vi "SwerveDriveRotate.vi"(7 "Trigger Axes":cluster{"Left":dbl, "Right":dbl}, 8 "error in (no error)":errorcluster, 9 "Center of Rotation Joystick Axes":cluster{"X":dbl, "Y":dbl}, 10 "Strafe Joystick Axes":cluster{"X":dbl, "Y":dbl}, 11 "Angle (degrees; 0 = right)":dbl) -> (0 "error out":errorcluster)   [LabVIEW 2014]
uses:
  Robot Global Data.vi
panel:
  out "FL":dbl(slide) scale=-1.0..1.0
  out "FR":dbl(slide) scale=-1.0..1.0
  out "RL":dbl(slide) scale=-1.0..1.0
  out "RR":dbl(slide) scale=-1.0..1.0
  out "RL":dbl(knob) scale=3.1416..-3.1416
  out "RR":dbl(knob) scale=3.1416..-3.1416
  out "FR":dbl(knob) scale=3.1416..-3.1416
  out "FL":dbl(knob) scale=3.1416..-3.1416
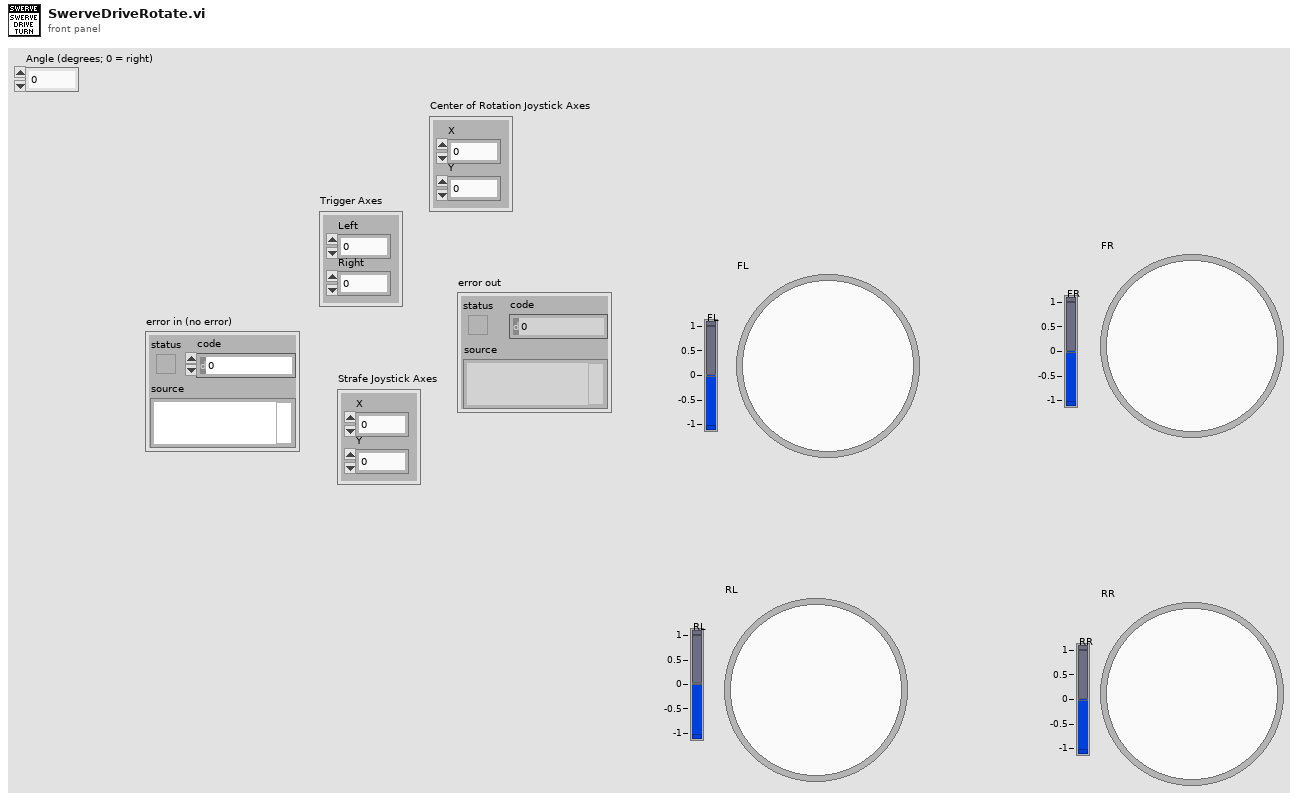
[diagram p1: front panel]
types:
  T1 = typedef "WPI_MotorControlDeviceRef.ctl" = cluster{"DeviceStatus":errorcluster, "Type":T2, "PWM":cluster{"Controller":T3, "PWM Channel":T4, "DeadBand":T5}, "CAN":cluster{"Device Number":u8, "Control Mode":T6, "Semaphore":T7, "Max Vout":dbl, "TalonSRX Control Mode":T8}, "Invert":bool, "TransformRef":T9, "InvTransformRef":T9}
  T2 = typedef "WPI_MotorControlType.ctl" = enum16{"PWM", "CAN", "CANTalonSRX"}
  T3 = typedef "FPGA_TypedefDigitalModule.ctl" = enum16{"Controller 1"}
  T4 = typedef "FPGA_DIOPWMChannel.ctl" = enum8{"PWM 0", "PWM 1", "PWM 2", "PWM 3", "PWM 4", "PWM 5", "PWM 6", "PWM 7", "PWM 8", "PWM 9", "PWM MXP 0", "PWM MXP 1", "PWM MXP 2", "PWM MXP 3", "PWM MXP 4", "PWM MXP 5", "PWM MXP 6", "PWM MXP 7", "PWM MXP 8", "PWM MXP 9", "Invalid"}
  T5 = typedef "WPI_PWMDeadband.ctl" = cluster{"Name":string, "maxPositivePwm":i32, "minPositivePwm":i32, "centerPwm":i32, "maxNegativePwm":i32, "minNegativePwm":i32, "angularRange":u16}
  T6 = typedef "WPI_CANJaguar_ControlMode.ctl" = enum8{"Percent VBus", "Current", "Speed", "Position", "Voltage"}
  T7 = typedef "Semaphore RefNum" = refnum<k1>
  T8 = typedef "WPI_CANTalonSRX_APIControlMode.ctl" = enum8{"Percent VBus", "Speed", "Position", "Slave", "Unchanged / Invalid"}
  T9 = typedef "WPI_PWMTransform_ConPane.ctl" = refnum<vi>
  T10 = typedef "WPI_CANTalonSRX_GlobalStatus.ctl" = cluster{"Applied Throttle":dbl, "Module Enabled":bool, "CAN Error":errorcluster, "Closed Loop Error":dbl, "Forward Limit Switch Closed":bool, "Reverse Limit Switch Closed":bool, "Sensor Position":dbl, "Sensor Velocity":dbl, "Current":dbl, "Sticky Fault - Over Temp":bool, "Sticky Fault - Under Voltage":bool, "Sticky Fault - Forward Limit":bool, "Sticky Fault - Reverse Limit":bool, "Sticky Fault - Forward Soft Limit":bool, "Sticky Fault - Reverse Soft Limit":bool, "Brake is Enabled":bool, "Encoder Position":dbl, "Encoder Velocity":dbl, "Encoder Index Count":dbl, "Encoder A Pin State":bool, "Encoder B Pin State":bool, "Encoder Index Pin State":bool, "Analog In":dbl, "Analog In Velocity":dbl, "Temperature (C)":dbl, "Battery Voltage":dbl}
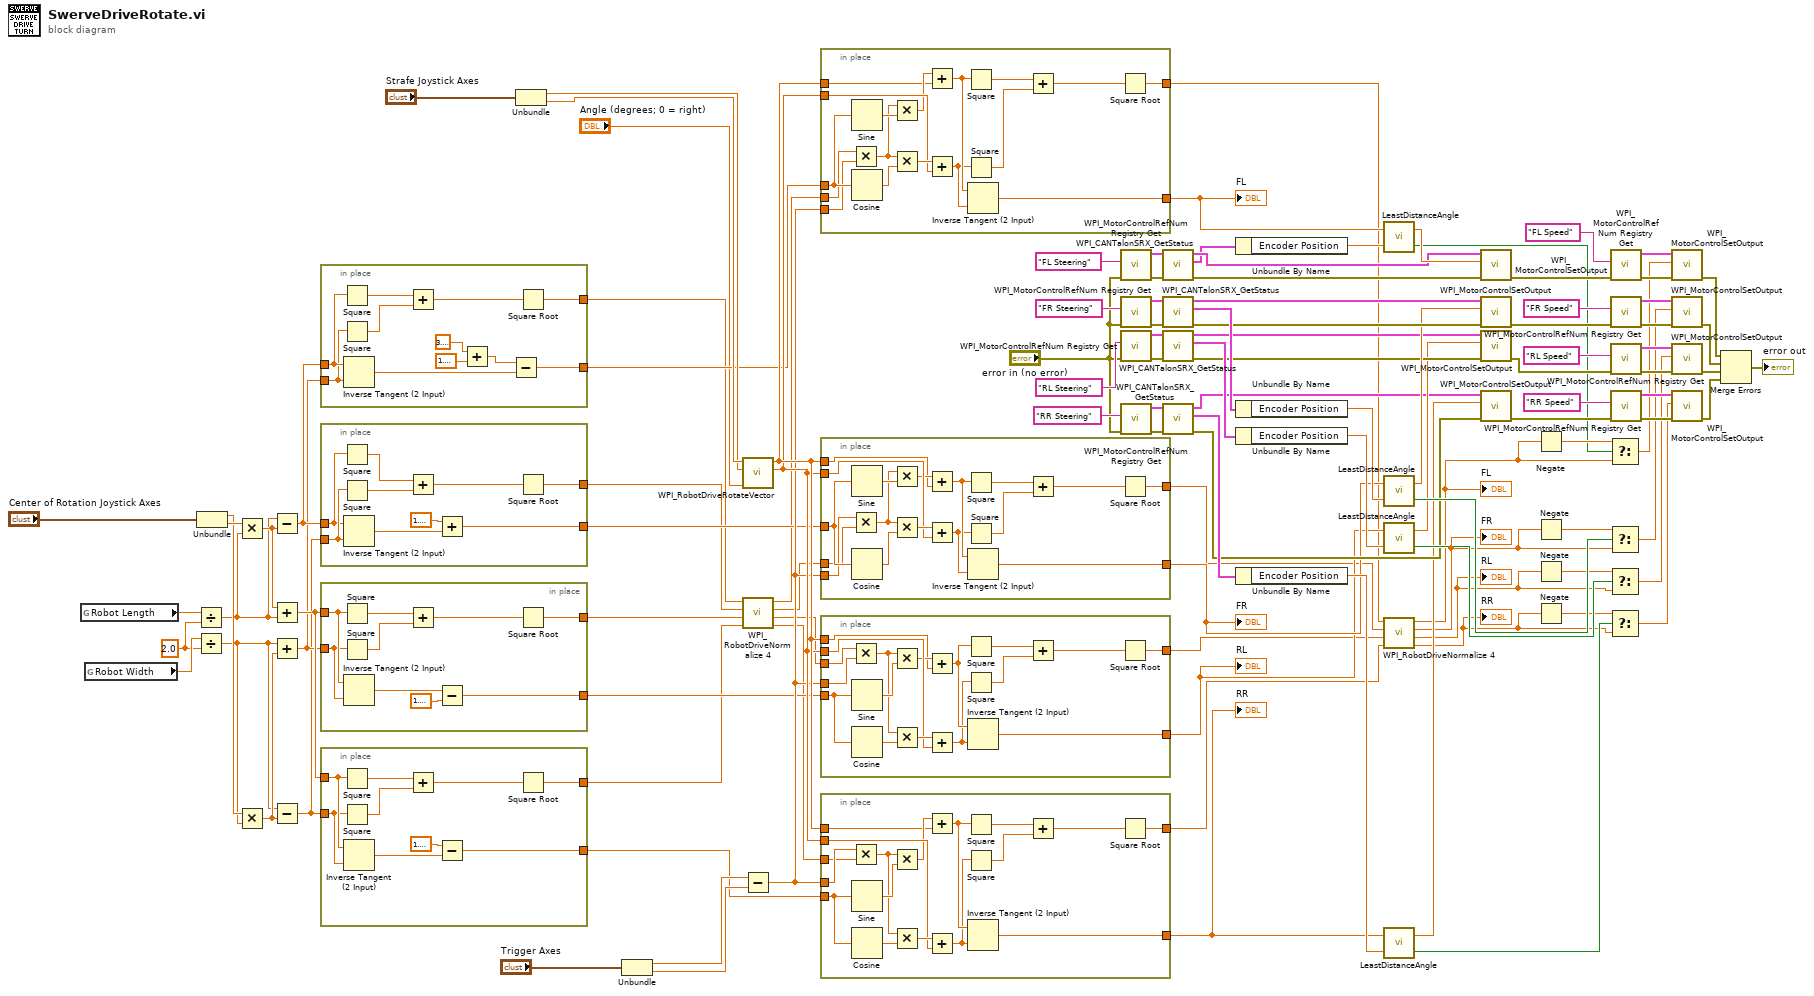
[diagram p0: block diagram]
diagram:
  w34 = 2.0 ("y")
  n1 = global read "Robot Global Data.vi" "Robot Length"() -> (w36:dbl)
  n2 = global read "Robot Global Data.vi" "Robot Width"() -> (w35:dbl)
  n3 = Divide(x=w36, y=w34) -> (x/y=w29:dbl)
  n4 = Divide(x=w35, y=w34) -> (x/y=w28:dbl)
  n5 = Unbundle("Center of Rotation Joystick Axes") -> ("X"=w32:dbl, "Y"=w33:dbl)
  n6 = Multiply(x=w33, y=w29) -> (x*y=w30:dbl)
  n7 = Multiply(x=w32, y=w28) -> (x*y=w31:dbl)
  n8 = Subtract(x=w29, y=w30) -> (x-y=w23:dbl)
  n9 = Add(x=w30, y=w29) -> (x+y=w22:dbl)
  n10 = Add(x=w28, y=w31) -> (x+y=w21:dbl)
  n11 = Subtract(x=w28, y=w31) -> (x-y=w19:dbl)
  n12 = in-place {
    in-place-border: [w125] -> w14
    in-place-border: w23 -> [w117]
    in-place-border: w21 -> [w116]
    in-place-border: [w115] -> w10
    n13 = Square(x=w117) -> (x^2=w119:dbl)
    n14 = Square(x=w116) -> (x^2=w118:dbl)
    n15 = Inverse Tangent (2 Input)(1:w116, 2:w117) -> (0:w121:dbl)
    n16 = Add(x=w119, y=w118) -> (x+y=w120:dbl)
    n17 = Add(x=3.141592653589793, y=1.5707963267948966) -> (x+y=w122:dbl)
    n18 = Subtract(x=w122, y=w121) -> (x-y=w125:dbl)
    n19 = Square Root(x=w120) -> (sqrt(x)=w115:dbl)
  }
  n20 = in-place {
    in-place-border: [w133] -> w13
    in-place-border: w19 -> [w128]
    in-place-border: w23 -> [w127]
    in-place-border: [w126] -> w8
    n21 = Square(x=w127) -> (x^2=w130:dbl)
    n22 = Square(x=w128) -> (x^2=w129:dbl)
    n23 = Inverse Tangent (2 Input)(1:w128, 2:w127) -> (0:w132:dbl)
    n24 = Add(x=w130, y=w129) -> (x+y=w131:dbl)
    n25 = Add(x=1.5707963267948966, y=w132) -> (x+y=w133:dbl)
    n26 = Square Root(x=w131) -> (sqrt(x)=w126:dbl)
  }
  n27 = in-place {
    in-place-border: [w142] -> w12
    in-place-border: w22 -> [w137]
    in-place-border: w21 -> [w136]
    in-place-border: [w135] -> w6
    n28 = Square(x=w137) -> (x^2=w139:dbl)
    n29 = Square(x=w136) -> (x^2=w138:dbl)
    n30 = Inverse Tangent (2 Input)(1:w136, 2:w137) -> (0:w141:dbl)
    n31 = Add(x=w139, y=w138) -> (x+y=w140:dbl)
    n32 = Subtract(x=w141, y=1.5707963267948966) -> (x-y=w142:dbl)
    n33 = Square Root(x=w140) -> (sqrt(x)=w135:dbl)
  }
  n34 = in-place {
    in-place-border: [w151] -> w11
    in-place-border: w22 -> [w146]
    in-place-border: w19 -> [w145]
    in-place-border: [w144] -> w4
    n35 = Square(x=w146) -> (x^2=w148:dbl)
    n36 = Square(x=w145) -> (x^2=w147:dbl)
    n37 = Inverse Tangent (2 Input)(1:w145, 2:w146) -> (0:w150:dbl)
    n38 = Add(x=w148, y=w147) -> (x+y=w149:dbl)
    n39 = Subtract(x=1.5707963267948966, y=w150) -> (x-y=w151:dbl)
    n40 = Square Root(x=w149) -> (sqrt(x)=w144:dbl)
  }
  n41 = Unbundle("Strafe Joystick Axes") -> ("X"=w101:dbl, "Y"=w102:dbl)
  n42 = Unbundle("Trigger Axes") -> ("Left"=w41:dbl, "Right"=w40:dbl)
  n43 = call <vilib>:"WPI_RobotDriveRotateVector.vi"("Angle"="Angle (degrees; 0 = right)", "X"=w101, "Y"=w102) -> ("X'"=w85:dbl, "Y'"=w86:dbl)  [unwired: 7 out]
  n44 = call <vilib>:"WPI_RobotDriveNormalize 4.vi"("D"=w4, "C"=w6, "B"=w8, "A"=w10) -> ("D'"=w3:dbl, "C'"=w5:dbl, "B'"=w7:dbl, "A'"=w9:dbl)
  n45 = Subtract(x=w41, y=w40) -> (x-y=w43:dbl)
  n46 = in-place {
    in-place-border: w14 -> [w164]
    in-place-border: w85 -> [w162]
    in-place-border: w86 -> [w160]
    in-place-border: [w157] -> w82
    in-place-border: w43 -> [w156]
    in-place-border: w9 -> [w155]
    in-place-border: [w154] -> w26
    n47 = Multiply(x=w155, y=w156) -> (x*y=w153:dbl)
    n48 = Sine(x=w164) -> (sin(x)=w166:dbl)
    n49 = Cosine(x=w164) -> (cos(x)=w165:dbl)
    n50 = Multiply(x=w153, y=w166) -> (x*y=w161:dbl)
    n51 = Multiply(x=w153, y=w165) -> (x*y=w163:dbl)
    n52 = Add(x=w161, y=w160) -> (x+y=w159:dbl)
    n53 = Add(x=w163, y=w162) -> (x+y=w158:dbl)
    n54 = Square(x=w159) -> (x^2=w168:dbl)
    n55 = Square(x=w158) -> (x^2=w167:dbl)
    n56 = Inverse Tangent (2 Input)(1:w158, 2:w159) -> (0:w157:dbl)
    n57 = Add(x=w168, y=w167) -> (x+y=w169:dbl)
    n58 = Square Root(x=w169) -> (sqrt(x)=w154:dbl)
  }
  "FL" <- w82
  n59 = in-place {
    in-place-border: w13 -> [w181]
    in-place-border: w85 -> [w179]
    in-place-border: w86 -> [w177]
    in-place-border: [w174] -> w38
    in-place-border: w43 -> [w173]
    in-place-border: [w172] -> w25
    in-place-border: w7 -> [w171]
    n60 = Multiply(x=w173, y=w171) -> (x*y=w170:dbl)
    n61 = Sine(x=w181) -> (sin(x)=w183:dbl)
    n62 = Cosine(x=w181) -> (cos(x)=w182:dbl)
    n63 = Multiply(x=w170, y=w183) -> (x*y=w178:dbl)
    n64 = Multiply(x=w170, y=w182) -> (x*y=w180:dbl)
    n65 = Add(x=w178, y=w177) -> (x+y=w176:dbl)
    n66 = Add(x=w180, y=w179) -> (x+y=w175:dbl)
    n67 = Square(x=w176) -> (x^2=w185:dbl)
    n68 = Square(x=w175) -> (x^2=w184:dbl)
    n69 = Inverse Tangent (2 Input)(1:w175, 2:w176) -> (0:w174:dbl)
    n70 = Add(x=w185, y=w184) -> (x+y=w186:dbl)
    n71 = Square Root(x=w186) -> (sqrt(x)=w172:dbl)
  }
  "FR" <- w38
  n72 = in-place {
    in-place-border: w85 -> [w197]
    in-place-border: w86 -> [w195]
    in-place-border: [w192] -> w37
    in-place-border: w43 -> [w191]
    in-place-border: w12 -> [w190]
    in-place-border: w5 -> [w188]
    in-place-border: [w187] -> w20
    n73 = Multiply(x=w188, y=w191) -> (x*y=w189:dbl)
    n74 = Sine(x=w190) -> (sin(x)=w200:dbl)
    n75 = Cosine(x=w190) -> (cos(x)=w199:dbl)
    n76 = Multiply(x=w189, y=w200) -> (x*y=w196:dbl)
    n77 = Multiply(x=w189, y=w199) -> (x*y=w198:dbl)
    n78 = Add(x=w196, y=w195) -> (x+y=w194:dbl)
    n79 = Add(x=w198, y=w197) -> (x+y=w193:dbl)
    n80 = Square(x=w194) -> (x^2=w202:dbl)
    n81 = Square(x=w193) -> (x^2=w201:dbl)
    n82 = Inverse Tangent (2 Input)(1:w193, 2:w194) -> (0:w192:dbl)
    n83 = Add(x=w202, y=w201) -> (x+y=w203:dbl)
    n84 = Square Root(x=w203) -> (sqrt(x)=w187:dbl)
  }
  "RL" <- w37
  n85 = in-place {
    in-place-border: w85 -> [w214]
    in-place-border: w86 -> [w212]
    in-place-border: [w209] -> w27
    in-place-border: w43 -> [w208]
    in-place-border: w11 -> [w207]
    in-place-border: w3 -> [w206]
    in-place-border: [w205] -> w24
    n86 = Multiply(x=w208, y=w206) -> (x*y=w204:dbl)
    n87 = Sine(x=w207) -> (sin(x)=w217:dbl)
    n88 = Cosine(x=w207) -> (cos(x)=w216:dbl)
    n89 = Multiply(x=w204, y=w217) -> (x*y=w213:dbl)
    n90 = Multiply(x=w204, y=w216) -> (x*y=w215:dbl)
    n91 = Add(x=w213, y=w212) -> (x+y=w211:dbl)
    n92 = Add(x=w215, y=w214) -> (x+y=w210:dbl)
    n93 = Square(x=w211) -> (x^2=w219:dbl)
    n94 = Square(x=w210) -> (x^2=w218:dbl)
    n95 = Inverse Tangent (2 Input)(1:w210, 2:w211) -> (0:w209:dbl)
    n96 = Add(x=w219, y=w218) -> (x+y=w220:dbl)
    n97 = Square Root(x=w220) -> (sqrt(x)=w205:dbl)
  }
  "RR" <- w27
  n98 = call <vilib>:"WPI_MotorControlRefNum Registry Get.vi"("error in (no error)"="error in (no error)", "refnum name"="FL Steering") -> ("error out"=w80:errorcluster, "MotorControlDevRef"=w112:T1)  [unwired: 8 in]
  n99 = call <vilib>:"WPI_MotorControlRefNum Registry Get.vi"("error in (no error)"="error in (no error)", "refnum name"="FR Steering") -> ("error out"=w68:errorcluster, "MotorControlDevRef"=w69:T1)  [unwired: 8 in]
  n100 = call <vilib>:"WPI_MotorControlRefNum Registry Get.vi"("error in (no error)"="error in (no error)", "refnum name"="RL Steering") -> ("error out"=w56:errorcluster, "MotorControlDevRef"=w57:T1)  [unwired: 8 in]
  n101 = call <vilib>:"WPI_MotorControlRefNum Registry Get.vi"("error in (no error)"="error in (no error)", "refnum name"="RR Steering") -> ("error out"=w48:errorcluster, "MotorControlDevRef"=w49:T1)  [unwired: 8 in]
  n102 = call <vilib>:"WPI_CANTalonSRX_GetStatus.vi"("error in (no error)"=w80, "CAN Talon SRX Ref"=w112) -> ("error out"=w79:errorcluster, "Talon SRX Status"=w78:T10, "CAN Talon SRX Ref Out"=w81:T1)  [unwired: 7 in]
  n103 = call <vilib>:"WPI_CANTalonSRX_GetStatus.vi"("error in (no error)"=w68, "CAN Talon SRX Ref"=w69) -> ("error out"=w66:errorcluster, "Talon SRX Status"=w73:T10, "CAN Talon SRX Ref Out"=w67:T1)  [unwired: 7 in]
  n104 = call <vilib>:"WPI_CANTalonSRX_GetStatus.vi"("error in (no error)"=w56, "CAN Talon SRX Ref"=w57) -> ("error out"=w59:errorcluster, "Talon SRX Status"=w63:T10, "CAN Talon SRX Ref Out"=w58:T1)  [unwired: 7 in]
  n105 = call <vilib>:"WPI_CANTalonSRX_GetStatus.vi"("error in (no error)"=w48, "CAN Talon SRX Ref"=w49) -> ("error out"=w47:errorcluster, "Talon SRX Status"=w53:T10, "CAN Talon SRX Ref Out"=w46:T1)  [unwired: 7 in]
  n106 = Unbundle By Name(w78) -> ("Encoder Position"=w77:dbl)
  n107 = Unbundle By Name(w73) -> ("Encoder Position"=w72:dbl)
  n108 = Unbundle By Name(w63) -> ("Encoder Position"=w62:dbl)
  n109 = Unbundle By Name(w53) -> ("Encoder Position"=w52:dbl)
  n110 = call "LeastDistanceAngle.vi"("current angle (no limits)"=w77, "target angle (between pi and -pi)"=w82) -> ("Reverse?"=w74:bool, "motor output angle"=w83:dbl)
  n111 = call "LeastDistanceAngle.vi"("current angle (no limits)"=w72, "target angle (between pi and -pi)"=w38) -> ("Reverse?"=w70:bool, "motor output angle"=w64:dbl)
  n112 = call "LeastDistanceAngle.vi"("current angle (no limits)"=w62, "target angle (between pi and -pi)"=w37) -> ("Reverse?"=w60:bool, "motor output angle"=w55:dbl)
  n113 = call <vilib>:"WPI_RobotDriveNormalize 4.vi"("D"=w24, "C"=w20, "B"=w25, "A"=w26) -> ("D'"=w15:dbl, "C'"=w16:dbl, "B'"=w18:dbl, "A'"=w17:dbl)
  "RR" <- w15
  "RL" <- w16
  "FR" <- w18
  "FL" <- w17
  n114 = call "LeastDistanceAngle.vi"("current angle (no limits)"=w52, "target angle (between pi and -pi)"=w27) -> ("Reverse?"=w50:bool, "motor output angle"=w45:dbl)
  n115 = call <vilib>:"WPI_MotorControlSetOutput.vi"("error in (no error)"=w79, "Output"=w83, "MotorControlDevRef"=w81) -> ("error out"=w109:errorcluster)  [unwired: 6 in, 2 out]
  n116 = call <vilib>:"WPI_MotorControlSetOutput.vi"("error in (no error)"=w66, "Output"=w64, "MotorControlDevRef"=w67) -> ("error out"=w104:errorcluster)  [unwired: 6 in, 2 out]
  n117 = call <vilib>:"WPI_MotorControlSetOutput.vi"("error in (no error)"=w59, "Output"=w55, "MotorControlDevRef"=w58) -> ("error out"=w93:errorcluster)  [unwired: 6 in, 2 out]
  n118 = call <vilib>:"WPI_MotorControlSetOutput.vi"("error in (no error)"=w47, "Output"=w45, "MotorControlDevRef"=w46) -> ("error out"=w87:errorcluster)  [unwired: 6 in, 2 out]
  n119 = Negate(x=w17) -> (-x=w75:dbl)
  n120 = Negate(x=w18) -> (-x=w71:dbl)
  n121 = Negate(x=w16) -> (-x=w61:dbl)
  n122 = Negate(x=w15) -> (-x=w51:dbl)
  n123 = Select(t=w75, s=w74, f=w17) -> (s? t:f=w76:dbl)
  n124 = Select(t=w71, s=w70, f=w18) -> (s? t:f=w65:dbl)
  n125 = Select(t=w61, s=w60, f=w16) -> (s? t:f=w54:dbl)
  n126 = Select(t=w51, s=w50, f=w15) -> (s? t:f=w44:dbl)
  n127 = call <vilib>:"WPI_MotorControlRefNum Registry Get.vi"("error in (no error)"=w109, "refnum name"="FL Speed") -> ("error out"=w111:errorcluster, "MotorControlDevRef"=w110:T1)  [unwired: 8 in]
  n128 = call <vilib>:"WPI_MotorControlRefNum Registry Get.vi"("error in (no error)"=w104, "refnum name"="FR Speed") -> ("error out"=w106:errorcluster, "MotorControlDevRef"=w105:T1)  [unwired: 8 in]
  n129 = call <vilib>:"WPI_MotorControlRefNum Registry Get.vi"("error in (no error)"=w93, "refnum name"="RL Speed") -> ("error out"=w95:errorcluster, "MotorControlDevRef"=w94:T1)  [unwired: 8 in]
  n130 = call <vilib>:"WPI_MotorControlRefNum Registry Get.vi"("error in (no error)"=w87, "refnum name"="RR Speed") -> ("error out"=w89:errorcluster, "MotorControlDevRef"=w88:T1)  [unwired: 8 in]
  n131 = call <vilib>:"WPI_MotorControlSetOutput.vi"("error in (no error)"=w111, "Output"=w76, "MotorControlDevRef"=w110) -> ("error out"=w98:errorcluster)  [unwired: 6 in, 2 out]
  n132 = call <vilib>:"WPI_MotorControlSetOutput.vi"("error in (no error)"=w106, "Output"=w65, "MotorControlDevRef"=w105) -> ("error out"=w100:errorcluster)  [unwired: 6 in, 2 out]
  n133 = call <vilib>:"WPI_MotorControlSetOutput.vi"("error in (no error)"=w95, "Output"=w54, "MotorControlDevRef"=w94) -> ("error out"=w92:errorcluster)  [unwired: 6 in, 2 out]
  n134 = call <vilib>:"WPI_MotorControlSetOutput.vi"("error in (no error)"=w89, "Output"=w44, "MotorControlDevRef"=w88) -> ("error out"=w84:errorcluster)  [unwired: 6 in, 2 out]
  n135 = Merge Errors(w98, w100, w92, w84) -> (→"error out":errorcluster)
